vi "build_time_arrays.vi"(10 "Delays":T1(array[cluster])) -> (2 "Array":dbl[](array[numeric]), 3 "ok":bool)   [LabVIEW 2015]
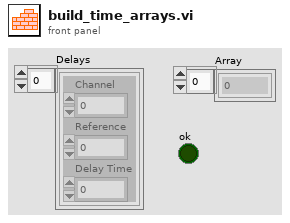
[diagram p1: front panel]
types:
  T1 = cluster{"Channel":u16, "Reference":u16, "Delay Time":dbl}[]
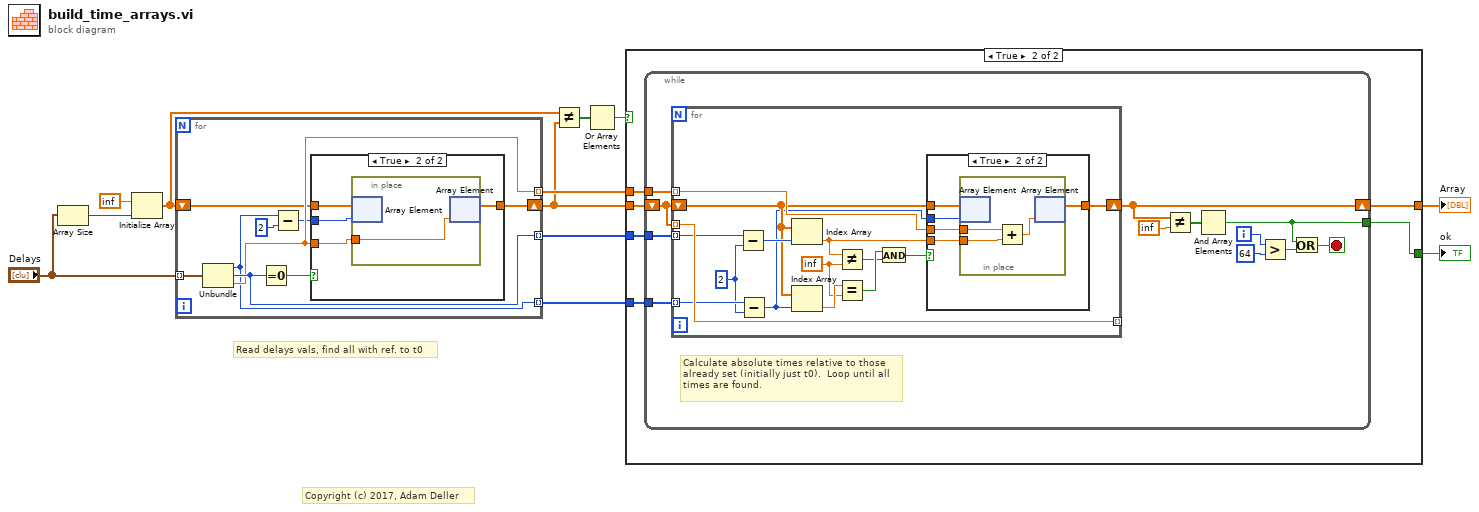
[diagram p0: block diagram]
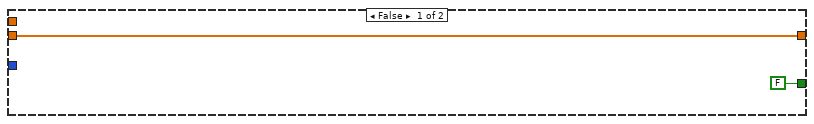
[diagram p2: hidden frame]
diagram:
  # "Copyright (c) 2017, Adam Deller"
  # "Read delays vals, find all with ref. to t0"
  n1 = Array Size(array="Delays") -> (size(s)=w12:i32)
  n2 = Initialize Array(inf, w12) -> (w7:dbl[])
  n3 = for {
    tunnel: "Delays" -> [w21] mode=indexing
    tunnel: [w18] -> w8 mode=indexing
    tunnel: [w20] -> w10 mode=indexing
    tunnel: [w15] -> w9 mode=indexing
    shift-right: [w19] -> w6
    shift-left: w7 -> [w16]
    n4 = Unbundle(w21) -> ("Channel"=w15:u16, "Reference"=w20:u16, "Delay Time"=w18:dbl)
    n5 = Equal To 0?(x=w20) -> (x = 0?=w17:bool)
    n6 = Subtract(x=w15, y=u16 2) -> (x-y=w13:u16)
    n7 = case shown="True" w17 {
      tunnel: w16 -> [w22 w26]
      tunnel: [w22 w25] -> w19
      tunnel: w18 -> [_ w24]
      tunnel: w13 -> [_ w23]
      frame False {
      }
      frame True {
        n8 = in-place {
          in-place-border: w24 -> [w27]
          n9 = in-place-array #1(w26, w23) -> ()  [unwired: 1 out]
          n10 = in-place-array #1(w27) -> (w25:dbl[])  [unwired: 1 out]
        }
      }
    }
  }
  n11 = Not Equal?(x=w7, y=w6) -> (x != y?=w5:bool[])
  n12 = Or Array Elements(Boolean array=w5) -> (logical OR=w4:bool)
  n13 = case shown="True" w4 {
    tunnel: w10 -> [_ w35]
    tunnel: w9 -> [_ w34]
    tunnel: w8 -> [_ w33]
    tunnel: [w28 w32] -> w2
    tunnel: [FALSE w31] -> w1
    tunnel: w6 -> [w28 w30]
    frame False {
    }
    frame True {
      n14 = while {
        shift-right: [w44] -> w32
        shift-left: w30 -> [w47]
        tunnel: w35 -> [w43]
        tunnel: w34 -> [w42]
        tunnel: w33 -> [w41]
        tunnel: [w37] -> w31
        i -> [w40]
        stop <- w38 stop-if-true
        # "Calculate absolute times relative to those\nalready set (initially just t0).  Loop until all\ntimes are found."
        n15 = for {
          tunnel: w47 -> [w62] mode=indexing
          tunnel: [w62] -> _ mode=indexing
          shift-right: [w55] -> w44
          shift-left: w47 -> [w54]
          tunnel: w43 -> [w61] mode=indexing
          tunnel: w42 -> [w59] mode=indexing
          tunnel: w41 -> [w56] mode=indexing
          w51 = inf
          w58 = u16 2 ("y")
          n16 = Subtract(x=w61, y=w58) -> (x-y=w60:u16)
          n17 = Subtract(x=w59, y=w58) -> (x-y=w53:u16)
          n18 = Index Array(array=w54, index=w60) -> (element=w57:dbl)
          n19 = Index Array(array=w54, index=w53) -> (element=w52:dbl)
          n20 = Not Equal?(x=w57, y=w51) -> (x != y?=w49:bool)
          n21 = Equal?(x=w52, y=w51) -> (x = y?=w50:bool)
          n22 = And(x=w50, y=w49) -> (x .and. y?=w48:bool)
          n23 = case shown="True" w48 {
            tunnel: w54 -> [w63 w68]
            tunnel: w53 -> [_ w67]
            tunnel: w57 -> [_ w66]
            tunnel: w56 -> [_ w65]
            tunnel: [w63 w64] -> w55
            frame False {
            }
            frame True {
              n24 = in-place {
                in-place-border: w66 -> [w71]
                in-place-border: w65 -> [w70]
                n25 = in-place-array #2(w68, w67) -> ()  [unwired: 1 out]
                n26 = Add(x=w70, y=w71) -> (x+y=w69:dbl)
                n27 = in-place-array #2(w69) -> (w64:dbl[])  [unwired: 1 out]
              }
            }
          }
        }
        n28 = Not Equal?(x=w44, y=inf) -> (x != y?=w45:bool[])
        n29 = And Array Elements(Boolean array=w45) -> (logical AND=w37:bool)
        n30 = Greater?(x=w40, y=64) -> (0:w36:bool)
        n31 = Or(x=w37, y=w36) -> (x .or. y?=w38:bool)
      }
    }
  }
  "Array" <- w2
  "ok" <- w1
